vi "Alarme_Atmosferico.vi"(6 "Internal Dew Point":dbl, 8 "Dew Point":dbl, 9 "Humidity":dbl, 10 "Wind Speed":dbl, 11 "LEAF":i32) -> (3 "PUB alarme atmosferico":string)   [LabVIEW 2018]
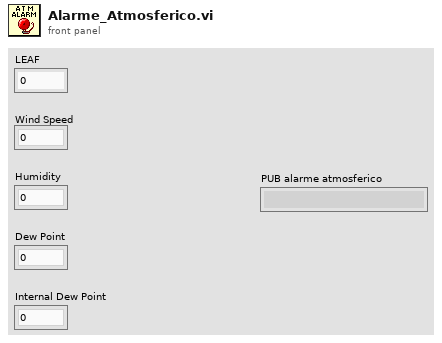
[diagram p1: front panel]
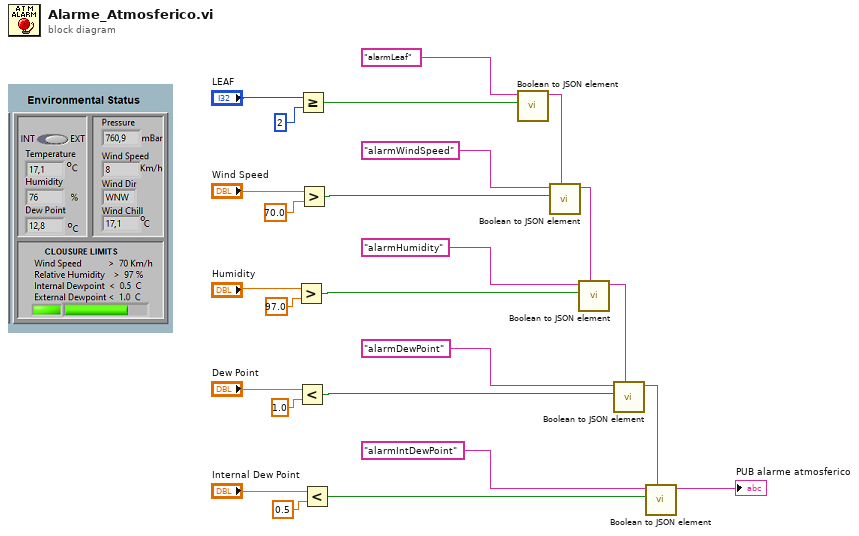
[diagram p0: block diagram]
diagram:
  n1 = Greater?(x="Humidity", y=97.0) -> (0:w6:bool)
  n2 = Less?(x="Dew Point", y=1.0) -> (x < y?=w4:bool)
  n3 = Greater Or Equal?(x="LEAF", y=2) -> (x >= y?=w9:bool)
  n4 = Greater?(x="Wind Speed", y=70.0) -> (0:w8:bool)
  n5 = Less?(x="Internal Dew Point", y=0.5) -> (x < y?=w2:bool)
  n6 = call "Boolean to JSON element.vi"("boolean"=w9, "keyword"="alarmLeaf") -> ("JSON element"=w7:string)  [unwired: 8 in, 1 out]
  n7 = call "Boolean to JSON element.vi"("prefix"=w7, "boolean"=w8, "keyword"="alarmWindSpeed") -> ("JSON element"=w5:string)  [unwired: 7 in, 1 out]
  n8 = call "Boolean to JSON element.vi"("prefix"=w5, "boolean"=w6, "keyword"="alarmHumidity") -> ("JSON element"=w3:string)  [unwired: 7 in, 1 out]
  n9 = call "Boolean to JSON element.vi"("prefix"=w3, "boolean"=w4, "keyword"="alarmDewPoint") -> ("JSON element"=w1:string)  [unwired: 7 in, 1 out]
  n10 = call "Boolean to JSON element.vi"("prefix"=w1, "boolean"=w2, "keyword"="alarmIntDewPoint") -> ("JSON element"=→"PUB alarme atmosferico":string)  [unwired: 7 in, 1 out]
